vi "global-rc-strings.vi"() -> ()   [LabVIEW 2020, in "CSMScript-Engine(Lite).lvlib"]
uses:
  CSMScript-Engine(Lite).lvlib
panel:
  in  "OI.ErrorDescription(Col4)":string="Error"
  in  "OI.TestStatus(Col3)":string="Status"
  in  "OI.StepIndex(Col0)":string
  in  "OI.TestResult(Col2)":string="Result"
  in  "OI.TestStep(Col1)":string="Step"
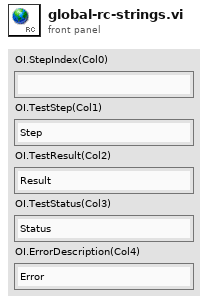
[diagram p1: front panel]
diagram:
